vi "TwoTanksModel_RealTime.vi"() -> ()   [LabVIEW 2016]
uses:
  <vilib>/Platform/TimedLoop/XDataNode/timing_clust.ctl
  <vilib>/Platform/TimedLoop/XDataNode/nitl_modes.ctl
  <vilib>/Platform/TimedLoop/XDataNode/wakeup.ctl
  <vilib>/Platform/TimedLoop/XDataNode/XDataNode.xnode
  <vilib>/Platform/TimedLoop/XDataNode/XDNodeRunTimeDep.lvlib
panel:
  out "H2 [cm]":dbl
  out "H1 [cm]":dbl
  in  "Valve2 On/Off":bool
  in  "Valve1 On/Off":bool
  in  "Pump On/Off":bool
  in  "stop":bool
  out "Waveform Chart":cluster{"H [cm]":dbl, "H [cm]":dbl}(graph)
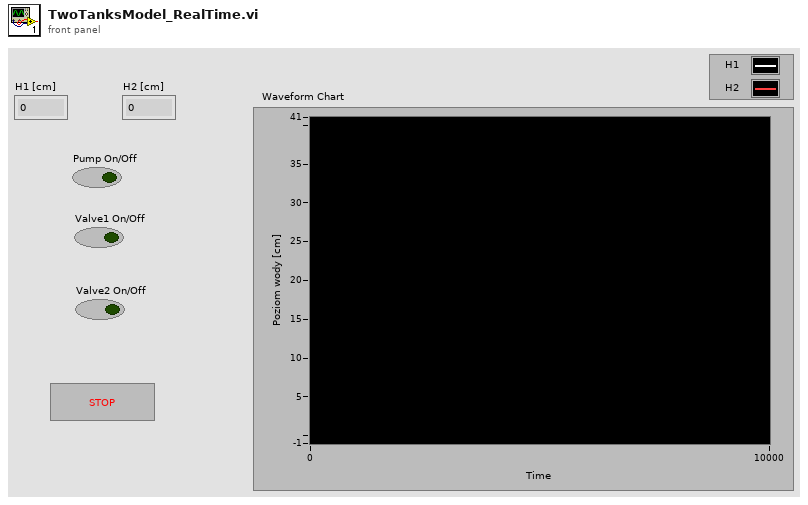
[diagram p1: front panel]
types:
  T1 = typedef "XDNodeRunTimeDep.lvlib/timing_clust.ctl" = cluster{"Expected End [f-1]":u64, "Actual End [f-1]":u64, "Finished Late? [f-1]":bool, "Expected End [i-1]":u64, "Actual End [i-1]":u64, "Finished Late? [i-1]":bool, "Expected Start [i]":u64, "Actual Start [i]":u64, "Expected Start [f]":u64, "Actual Start [f]":u64, "Source Name":string, "Structure Name":string, "Period":i64, "Deadline":i64, "Offset":i64, "Start":i64, "Priority":i32, "Timeout":i32, "Mode":T2, "Wakeup Reason":T3, "Error":errorcluster, "Source Type":string, "Secondary Source Type":string, "Global End Time":u64, "Global Start Time":u64, "Frame Duration":u64, "Iteration Duration":u64, "Assigned CPU":i32, "I/O Scan Engine Mode":u32}
  T2 = typedef "XDNodeRunTimeDep.lvlib/nitl_modes.ctl" = enum32{"No Change", "Process missed periods, maintain original phase", "Discard missed periods, maintain original phase", "Process missed periods, ignore original phase", "Discard missed periods, ignore original phase"}
  T3 = typedef "XDNodeRunTimeDep.lvlib/wakeup.ctl" = enum32{"Normal", "Aborted", "Asynchronous wakeup", "Timing source error", "Timed loop error", "Timeout"}
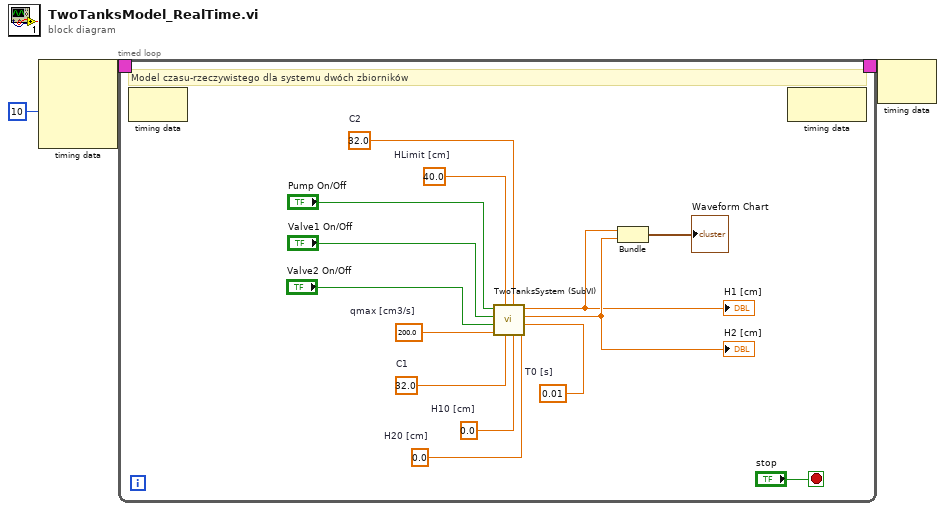
[diagram p0: block diagram]
diagram:
  n1 = node-c288(i64 10 ("Period")) -> (w3:T1)  [unwired: 3 in]
  n2 = timed-loop {
    timing: w3 -> [_]
    timing-out: [_] -> w2
    stop <- "stop" stop-if-true
    w15 = 0.01  # T0 [s]
    w4 = 32.0  # C2
    w10 = 32.0  # C1
    w12 = 0.0  # H20 [cm]
    w11 = 0.0  # H10 [cm]
    w5 = 40.0  # HLimit [cm]
    w9 = 200.0  # qmax [cm3/s]
    # "Model czasu-rzeczywistego dla systemu dwóch zbiorników"
    n3 = node-c288() -> ()  [unwired: 1 in, 1 out]
    n4 = call "TwoTanksSystem (SubVI).vi"("H20 [cm]"=w12, "T0 [s]"=w15, "H10 [cm]"=w11, "C2"=w4, "C1"=w10, "HLimit [cm]"=w5, "qmax [cm3/s]"=w9, "Valve2 On/Off"="Valve2 On/Off", "Valve1 On/Off"="Valve1 On/Off", "Pump On/Off"="Pump On/Off") -> ("H2 [cm]"=w14:dbl, "H1 [cm]"=w13:dbl)
    "H1 [cm]" <- w13
    "H2 [cm]" <- w14
    n5 = Bundle("H1 [cm]"=w13, "H2 [cm]"=w14) -> (→"Waveform Chart":cluster{"H1 [cm]":dbl, "H2 [cm]":dbl})  [unwired: 1 in]
    n6 = node-c288() -> ()  [unwired: 1 in, 1 out]
  }
  n7 = node-c288(w2) -> ()  [unwired: 1 out]
